vi "Convert Trace to CAN Frame.vi"(11 "captured data in":string[][](array[string])) -> (2 "can frames out":T1[](array[typedef]) {"payload" format="%x"; "timestamp" format="%<%.7X\n%x>T"; "type" items=["CAN Data"=0, "CAN Remote"=1, "CAN Bus Error"=2, "CAN 2.0 Data"=8, "CAN FD Data"=16, "CAN FD+BRS Data"=24, "J1939 Data"=192, "Delay"=224, "Log Trigger"=225, "Start Trigger"=226]; "identifier" format="%x"})   [LabVIEW 2025, in "CAN-LIN Raw Bus Capture UI.lvlib"]
uses:
  CAN-LIN Raw Bus Capture UI.lvlib
  <vilib>/xnet/xnet.llb/XNET Frame CAN.ctl
  <vilib>/xnet/xnet.llb/XNET Frame Type CAN.ctl
panel:
  in  "payload":u8[](array[numeric])
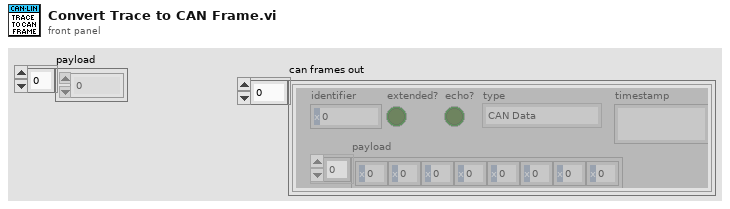
[diagram p1: front panel]
types:
  T1 = typedef "XNET Frame CAN.ctl" = cluster{"timestamp":timestamp, "payload":u8[], "identifier":u32, "type":T2, "extended?":bool, "echo?":bool}
  T2 = typedef "XNET Frame Type CAN.ctl" = u8
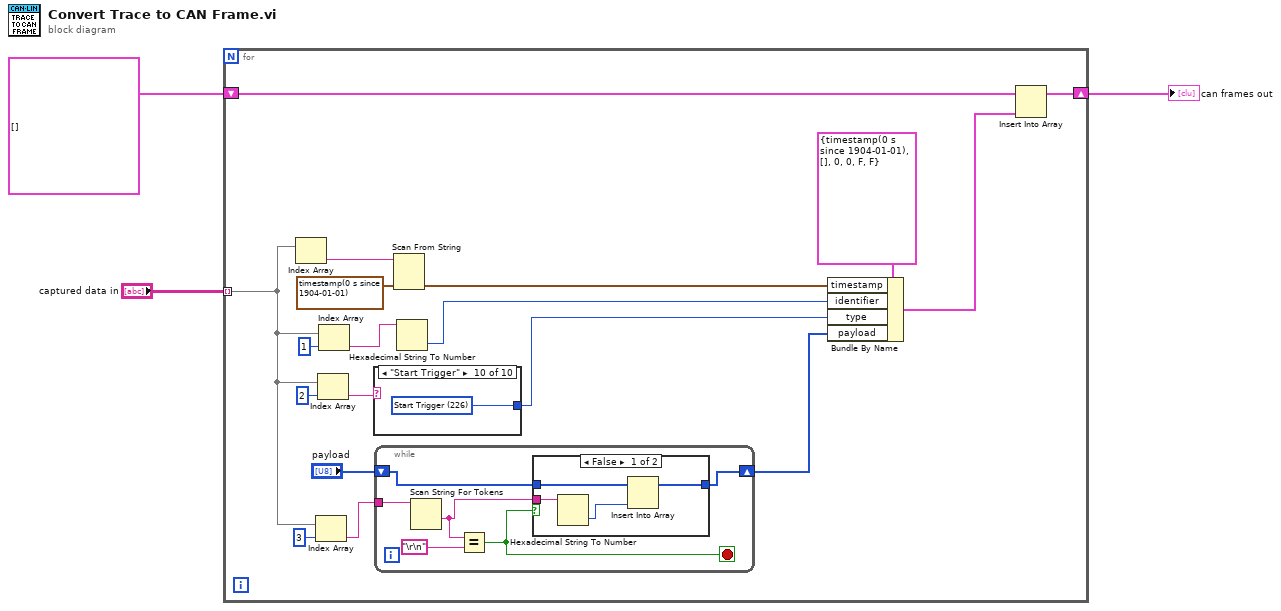
[diagram p0: block diagram]
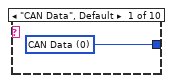
[diagram p3: hidden frame]
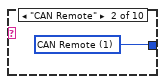
[diagram p4: hidden frame]
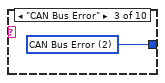
[diagram p5: hidden frame]
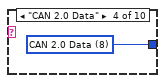
[diagram p6: hidden frame]
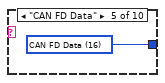
[diagram p7: hidden frame]
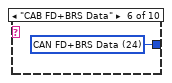
[diagram p8: hidden frame]
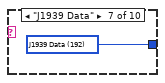
[diagram p9: hidden frame]
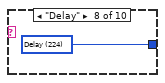
[diagram p10: hidden frame]
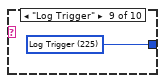
[diagram p11: hidden frame]
diagram:
  n1 = for {
    tunnel: "captured data in" -> [w8] mode=indexing
    shift-right: [w18] -> w1
    shift-left: T1[] [] ("CAN frames") -> [w19]
    n2 = Index Array(array=w8) -> (element=w16:string)  [unwired: 1 in]
    n3 = Index Array(array=w8, index=3) -> (element=w6:string)
    n4 = Index Array(array=w8, index=2) -> (element=w10:string)
    n5 = Index Array(array=w8, index=1) -> (element=w13:string)
    n6 = case shown="\"Start Trigger\"" w10 {
      tunnel: [w33 w34 w35 w36 w37 w38 w39 w40 w41 w42] -> w9
      frame "CAN Data", Default {
        w33 = T2 0 items=["CAN Data"=0, "CAN Remote"=1, "CAN Bus Error"=2, "CAN 2.0 Data"=8, "CAN FD Data"=16, "CAN FD+BRS Data"=24, "J1939 Data"=192, "Delay"=224, "Log Trigger"=225, "Start Trigger"=226] ("type")
      }
      frame "CAN Remote" {
        w34 = T2 1 items=["CAN Data"=0, "CAN Remote"=1, "CAN Bus Error"=2, "CAN 2.0 Data"=8, "CAN FD Data"=16, "CAN FD+BRS Data"=24, "J1939 Data"=192, "Delay"=224, "Log Trigger"=225, "Start Trigger"=226] ("type")
      }
      frame "CAN Bus Error" {
        w35 = T2 2 items=["CAN Data"=0, "CAN Remote"=1, "CAN Bus Error"=2, "CAN 2.0 Data"=8, "CAN FD Data"=16, "CAN FD+BRS Data"=24, "J1939 Data"=192, "Delay"=224, "Log Trigger"=225, "Start Trigger"=226] ("type")
      }
      frame "CAN 2.0 Data" {
        w36 = T2 8 items=["CAN Data"=0, "CAN Remote"=1, "CAN Bus Error"=2, "CAN 2.0 Data"=8, "CAN FD Data"=16, "CAN FD+BRS Data"=24, "J1939 Data"=192, "Delay"=224, "Log Trigger"=225, "Start Trigger"=226] ("type")
      }
      frame "CAN FD Data" {
        w37 = T2 16 items=["CAN Data"=0, "CAN Remote"=1, "CAN Bus Error"=2, "CAN 2.0 Data"=8, "CAN FD Data"=16, "CAN FD+BRS Data"=24, "J1939 Data"=192, "Delay"=224, "Log Trigger"=225, "Start Trigger"=226] ("type")
      }
      frame "CAB FD+BRS Data" {
        w38 = T2 24 items=["CAN Data"=0, "CAN Remote"=1, "CAN Bus Error"=2, "CAN 2.0 Data"=8, "CAN FD Data"=16, "CAN FD+BRS Data"=24, "J1939 Data"=192, "Delay"=224, "Log Trigger"=225, "Start Trigger"=226] ("type")
      }
      frame "J1939 Data" {
        w39 = T2 192 items=["CAN Data"=0, "CAN Remote"=1, "CAN Bus Error"=2, "CAN 2.0 Data"=8, "CAN FD Data"=16, "CAN FD+BRS Data"=24, "J1939 Data"=192, "Delay"=224, "Log Trigger"=225, "Start Trigger"=226] ("type")
      }
      frame "Delay" {
        w40 = T2 224 items=["CAN Data"=0, "CAN Remote"=1, "CAN Bus Error"=2, "CAN 2.0 Data"=8, "CAN FD Data"=16, "CAN FD+BRS Data"=24, "J1939 Data"=192, "Delay"=224, "Log Trigger"=225, "Start Trigger"=226] ("type")
      }
      frame "Log Trigger" {
        w41 = T2 225 items=["CAN Data"=0, "CAN Remote"=1, "CAN Bus Error"=2, "CAN 2.0 Data"=8, "CAN FD Data"=16, "CAN FD+BRS Data"=24, "J1939 Data"=192, "Delay"=224, "Log Trigger"=225, "Start Trigger"=226] ("type")
      }
      frame "Start Trigger" {
        w42 = T2 226 items=["CAN Data"=0, "CAN Remote"=1, "CAN Bus Error"=2, "CAN 2.0 Data"=8, "CAN FD Data"=16, "CAN FD+BRS Data"=24, "J1939 Data"=192, "Delay"=224, "Log Trigger"=225, "Start Trigger"=226] ("type")
      }
    }
    n7 = while {
      tunnel: w6 -> [w27]
      shift-right: [w23] -> w4
      shift-left: "payload" -> [w24]
      stop <- w25 stop-if-true
      n8 = Scan String For Tokens(9:w27) -> (1:w22:string)  [unwired: 5 in, 3 out]
      n9 = Equal?(x=w22, y="\r\n") -> (x = y?=w25:bool)
      n10 = case shown="False" w25 {
        tunnel: w24 -> [w30 w32]
        tunnel: [w28 w32] -> w23
        tunnel: w22 -> [w31 _]
        frame False {
          n11 = Hexadecimal String To Number(string=w31) -> (number=w29:u32)  [unwired: 2 in, 1 out]
          n12 = Insert Into Array(array=w30, new element=w29) -> (w28:u8[])  [unwired: 1 in]
        }
        frame True {
        }
      }
    }
    n13 = Scan From String(input string=w16, default 1=timestamp(0 s since 1904-01-01) ("timestamp")) -> (output 1=w15:timestamp)  [unwired: 3 in, 3 out]
    n14 = Hexadecimal String To Number(string=w13) -> (number=w12:u32)  [unwired: 2 in, 1 out]
    n15 = Bundle By Name(cluster=T1 {"timestamp"=timestamp(0 s since 1904-01-01), "payload"=[], "identifier"=0, "type"=0, "extended?"=FALSE, "echo?"=FALSE} ("CAN frame"), "timestamp"=w15, "identifier"=w12, "type"=w9, "payload"=w4) -> (w20:T1)
    n16 = Insert Into Array(array=w19, new element=w20) -> (w18:T1[])  [unwired: 1 in]
  }
  "can frames out" <- w1
